vi "VIs_for_All_Demos.vi"(8 "error in (no error)":errorcluster) -> (0 "error out":errorcluster, 3 "Strings []":string[](array[string]))   [LabVIEW 2011]
panel:
  in  "Listbox to change order (drag)":i32(listbox)
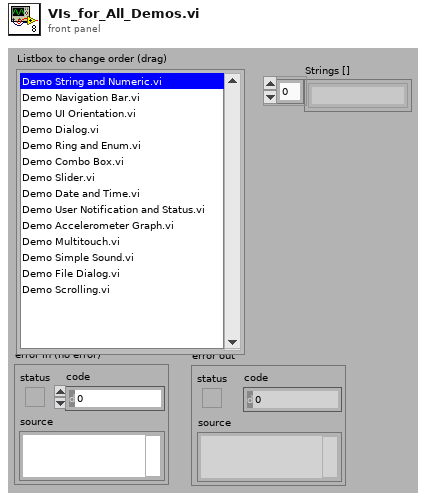
[diagram p1: front panel]
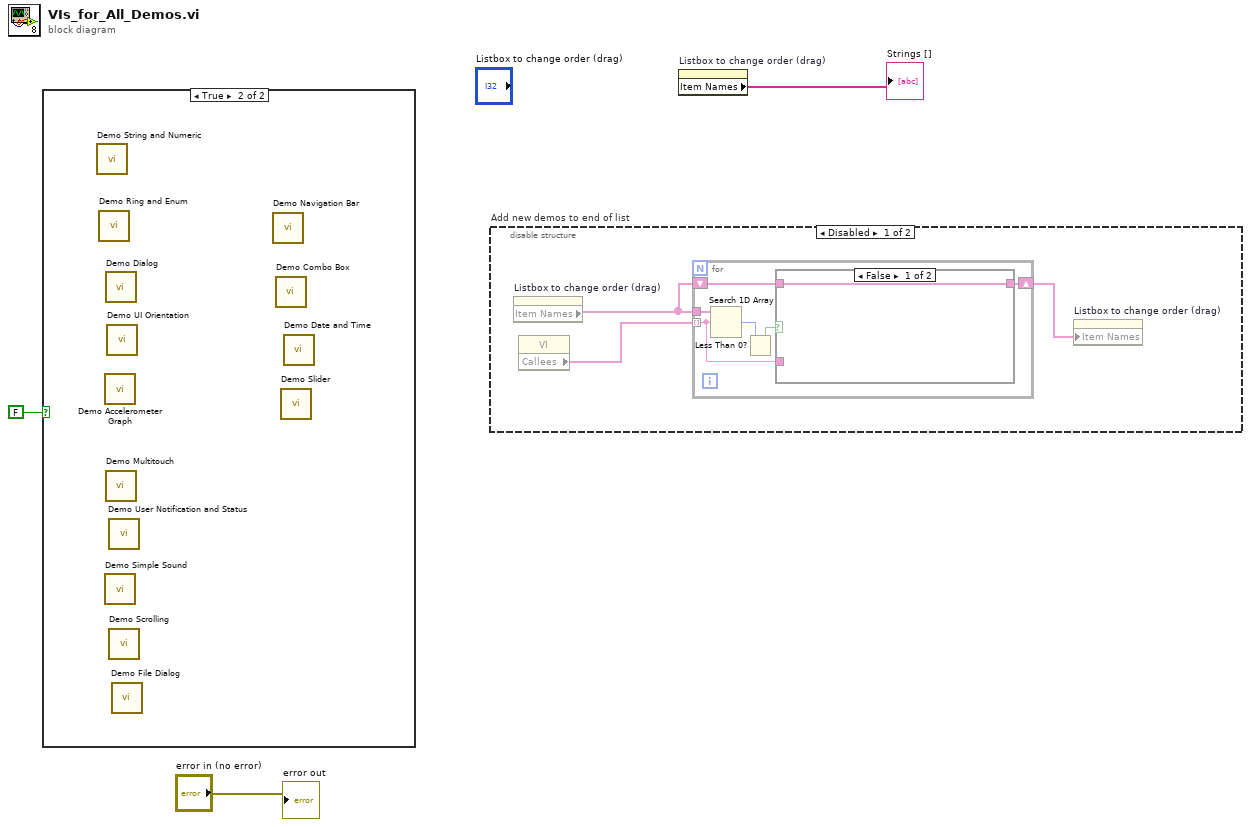
[diagram p0: block diagram]
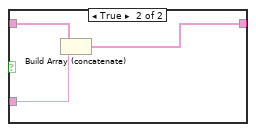
[diagram p2: hidden frame]
diagram:
  n1 = case shown="True" FALSE {
    frame False {
    }
    frame True {
      n2 = call "Demo String and Numeric.vi"() -> ()  [unwired: 1 in, 11 out]
      n3 = call "Demo Ring and Enum.vi"() -> ()  [unwired: 1 in, 11 out]
      n4 = call "Demo Accelerometer Graph.vi"() -> ()  [unwired: 1 in, 11 out]
      n5 = call "Demo Simple Sound.vi"() -> ()  [unwired: 1 in, 11 out]
      n6 = call "Demo Dialog.vi"() -> ()  [unwired: 1 in, 11 out]
      n7 = call "Demo Multitouch.vi"() -> ()  [unwired: 1 in, 11 out]
      n8 = call "Demo UI Orientation.vi"() -> ()  [unwired: 1 in, 11 out]
      n9 = call "Demo User Notification and Status.vi"() -> ()  [unwired: 1 in, 11 out]
      n10 = call "Demo Scrolling.vi"() -> ()  [unwired: 1 in, 11 out]
      n11 = call "Demo File Dialog.vi"() -> ()  [unwired: 1 in, 11 out]
      n12 = call "Demo Navigation Bar.vi"() -> ()  [unwired: 1 in, 11 out]
      n13 = call "Demo Combo Box.vi"() -> ()  [unwired: 1 in, 11 out]
      n14 = call "Demo Slider.vi"() -> ()  [unwired: 1 in, 11 out]
      n15 = call "Demo Date and Time.vi"() -> ()  [unwired: 1 in, 11 out]
    }
  }
  n16 = disable-structure "Add new demos to end of list" shown="Disabled" {
    frame Disabled {
      n17 = property on="Listbox to change order (drag)" class="LstBox (strict)"() -> ("Item Names"=w5:string[])  [unwired: 2 in, 2 out]
      n18 = property class="VI"() -> ("Callees"=w6:string[])  [unwired: 2 in, 2 out]
      n19 = for {
        tunnel: w5 -> [w12]
        tunnel: w6 -> [w8] mode=indexing
        shift-right: [w7] -> w4
        shift-left: w5 -> [w9]
        n20 = Search 1D Array(1D array=w12, element=w8) -> (index of element=w11:i32)  [unwired: 1 in]
        n21 = Less Than 0?(x=w11) -> (x < 0?=w10:bool)
        n22 = case shown="False" w10 {
          tunnel: w9 -> [w13 w16]
          tunnel: w8 -> [_ w15]
          tunnel: [w13 w14] -> w7
          frame False {
          }
          frame True {
            n23 = Build Array (concatenate)(w16, w15) -> (w14:string[])
          }
        }
      }
      n24 = property on="Listbox to change order (drag)" class="LstBox (strict)"("Item Names"=w4) -> ()  [unwired: 2 in, 2 out]
    }
    frame Enabled {
    }
  }
  n25 = property on="Listbox to change order (drag)" class="LstBox (strict)"() -> ("Item Names"=→"Strings []":string[])  [unwired: 2 in, 2 out]
  "error out" <- "error in (no error)"
